vi "Staging1Wire.vi"() -> ()   [LabVIEW 2013]
uses:
  Device Driver/1WireSystem/subVis/position_TypDef.ctl
  shared programs/GUI_Template/GUI_master/tcp new data cluster.ctl
panel:
  in  "Position.Channel 8::1":T1(ring) caption="Position.Channel 7::1"
  in  "Filpper.Channel 8.Name::1":string caption="Filpper.Channel 7.Name::1"
  in  "Position.Channel 1::1":T2
  in  "all out":bool
  in  "Beam1":bool
  in  "Beam2":bool
  in  "Filpper.Channel 7.Name::1":string
  in  "Position.Channel 7::1":T1(ring)
  in  "Position.Channel 6::1":T1(ring)
  in  "Filpper.Channel 6.Name::1":string
  in  "Position.Channel 5::1":T1(ring)
  in  "Filpper.Channel 5.Name::1":string="Beam2 Near"
  in  "Position.Channel 4::1":T1(ring)
  in  "Filpper.Channel 4.Name::1":string="Beam1 Far"
  in  "Filpper.Channel 3.Name::1":string="Beam1 Near"
  in  "Filpper.Channel 2.Name::1":string="Beam2 Far"
  in  "Position.Channel 3::1":T1(ring)
  in  "Filpper.Channel 1.Name::1":string="XH1"
  in  "Position.Channel 2::1":T1(ring)
  out "device status::1":string="Initialized"
  in  "stop":bool
  in  "GUIdevice 1":string="Staging1Wire"
  out "UDP error message":string
  in  "insert tag":bool=TRUE
  # "Staging 1Wire"
  # "Far"
  # "Near"
  # "Far"
  # "Near"
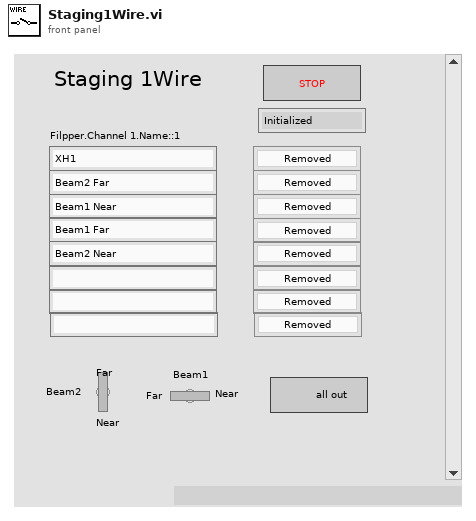
[diagram p1: front panel]
types:
  T1 = enum16{"Removed", "Inserted", "Unknown", "Moving"}
  T2 = typedef "position_TypDef.ctl" = enum16{"Removed", "Inserted", "Unknown", "Moving"}
  T3 = typedef "tcp new data cluster.ctl" = cluster{"EventEnum":enum16{"new data", "connection status update"}, "Device name":string}
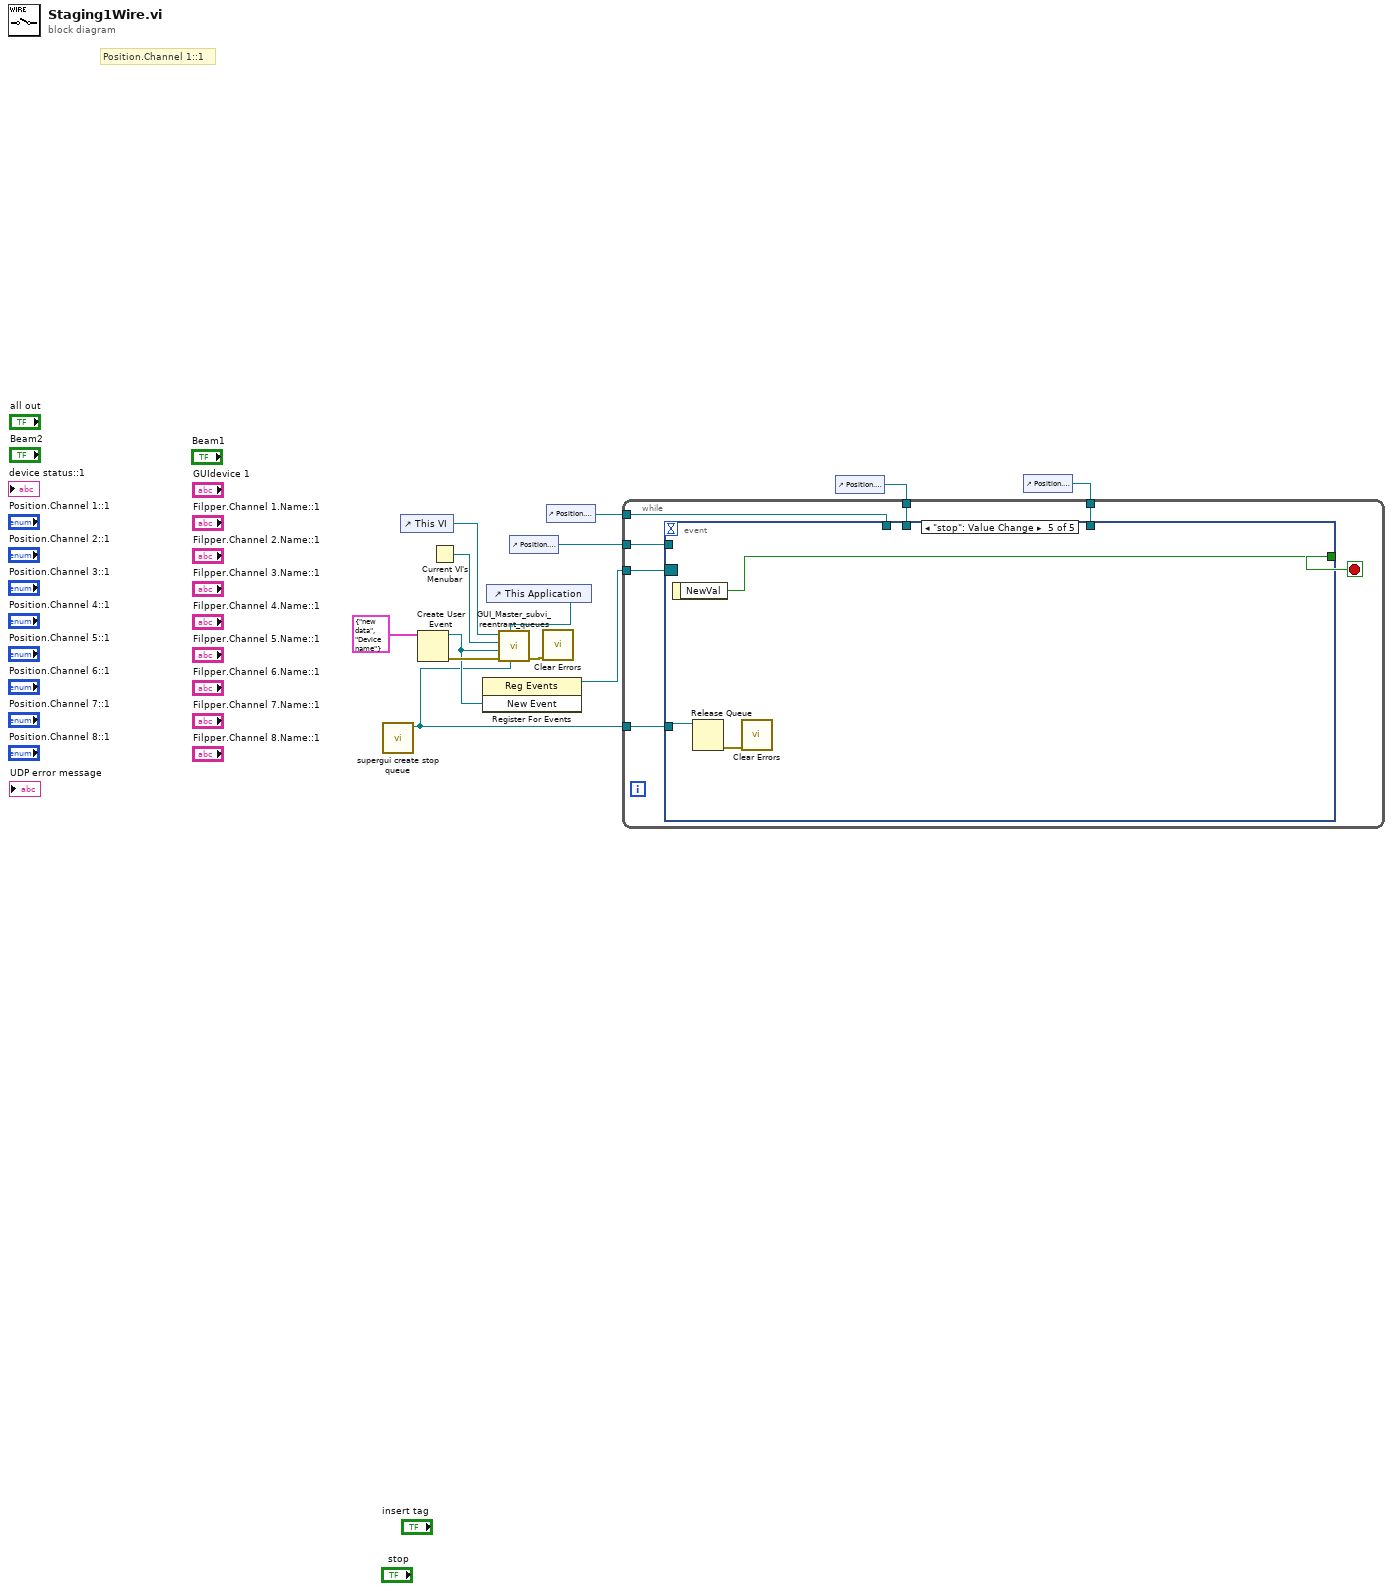
[diagram p0: block diagram]
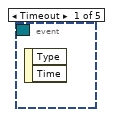
[diagram p2: hidden frame]
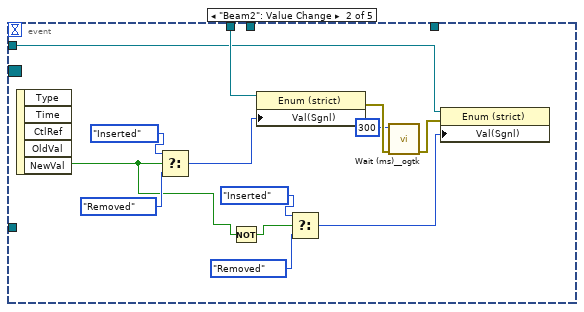
[diagram p3: hidden frame]
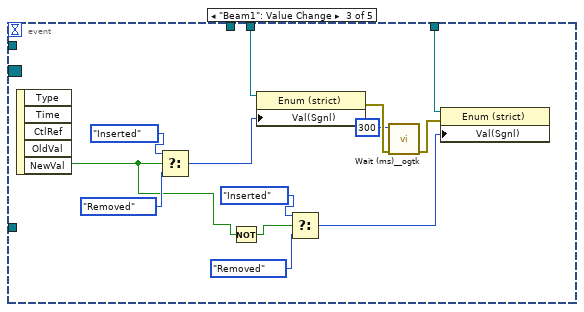
[diagram p4: hidden frame]
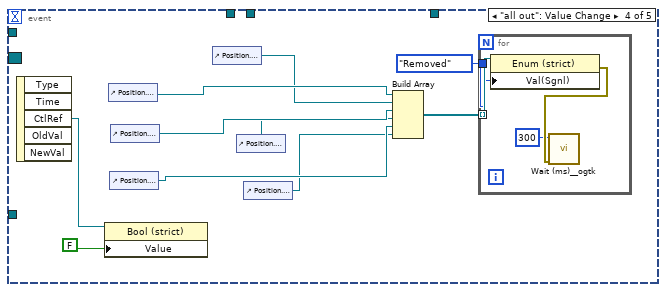
[diagram p5: hidden frame]
diagram:
  # "Position.Channel 1::1"
  n1 = call "supergui create stop queue.vi"() -> ("STOP Queue out"=w1:refnum<queue>)  [unwired: 11 in]
  n2 = control-ref of="This VI"() -> (w13:refnum<vi>)
  n3 = Create User Event(user event datatype=T3 {"EventEnum"=enum."new data", "Device name"="Device name"} ("New Event")) -> (user event=w8:refnum<user-event>, error out=w10:errorcluster)  [unwired: 1 in]
  n4 = Current VI's Menubar() -> (w12:refnum<k9>)
  n5 = register-events(w8) -> (reference out=w7:refnum<event-registration>)  [unwired: 2 in, 1 out]
  n6 = control-ref of="This Application"() -> (w2:refnum<vi>)
  n7 = call "GUI_Master_subvi_reentrant_queues.vi"("STOP Queue in"=w1, "This Application"=w2, "error in (no error)"=w10, "tcp data event"=w8, "Caller menu reference"=w12, "Caller VI ref"=w13) -> ("error out"=w9:errorcluster)  [unwired: 5 in]
  n8 = control-ref of="Position.Channel 5::1"() -> (w5:refnum<vi>)
  n9 = call <vilib>:"Clear Errors.vi"("error in (no error)"=w9) -> ()  [unwired: 6 in, 1 out]
  n10 = control-ref of="Position.Channel 2::1"() -> (w6:refnum<vi>)
  n11 = control-ref of="Position.Channel 3::1"() -> (w4:refnum<vi>)
  n12 = control-ref of="Position.Channel 4::1"() -> (w3:refnum<vi>)
  n13 = while {
    tunnel: w7 -> [w20]
    tunnel: w6 -> [w18]
    tunnel: w5 -> [w17]
    tunnel: w4 -> [w16]
    tunnel: w3 -> [w15]
    tunnel: w1 -> [w14]
    stop <- w19 stop-if-true
    n14 = event shown="[4] \"stop\": Value Change" {
      selector: w20 -> [_ _ _ _ _]
      dyn-events: _ -> [_ _ _ _ _]
      timeout: _ -> [_ _ _ _ _]
      tunnel: [_ _ _ _ w63] -> w19
      tunnel: w18 -> [_ w33 _ _ _]
      tunnel: w17 -> [_ w26 _ _ _]
      tunnel: w16 -> [_ _ w35 _ _]
      tunnel: w15 -> [_ _ w34 _ _]
      tunnel: w14 -> [_ _ _ _ w62]
      event Timeout {
        n15 = event-data() -> ()  [unwired: 1 in, 2 out]
      }
      event "Beam2": Value Change {
        n16 = event-data() -> ("NewVal"=w28:bool)  [unwired: 1 in, 4 out]
        n17 = Select(t=T1."Inserted" ("Value"), s=w28, f=T1."Removed" ("Value")) -> (s? t:f=w24:T1)
        n18 = Not(x=w28) -> (.not. x?=w27:bool)
        n19 = property class="Enum (strict)"(reference=w33, "Val(Sgnl)"=w24) -> (error out=w23:errorcluster)  [unwired: 1 in, 1 out]
        n20 = Select(t=T1."Inserted" ("Value"), s=w27, f=T1."Removed" ("Value")) -> (s? t:f=w25:T1)
        n21 = call <userlib>:"Wait (ms)__ogtk.vi"("error in (no error)"=w23, "milliseconds to wait"=u32 300) -> ("error out"=w22:errorcluster)  [unwired: 8 in, 1 out]
        n22 = property class="Enum (strict)"(reference=w26, error in=w22, "Val(Sgnl)"=w25) -> ()  [unwired: 2 out]
      }
      event "Beam1": Value Change {
        n23 = event-data() -> ("NewVal"=w42:bool)  [unwired: 1 in, 4 out]
        n24 = Select(t=T1."Inserted" ("Value"), s=w42, f=T1."Removed" ("Value")) -> (s? t:f=w39:T1)
        n25 = Not(x=w42) -> (.not. x?=w41:bool)
        n26 = property class="Enum (strict)"(reference=w35, "Val(Sgnl)"=w39) -> (error out=w38:errorcluster)  [unwired: 1 in, 1 out]
        n27 = Select(t=T1."Inserted" ("Value"), s=w41, f=T1."Removed" ("Value")) -> (s? t:f=w40:T1)
        n28 = call <userlib>:"Wait (ms)__ogtk.vi"("error in (no error)"=w38, "milliseconds to wait"=u32 300) -> ("error out"=w37:errorcluster)  [unwired: 8 in, 1 out]
        n29 = property class="Enum (strict)"(reference=w34, error in=w37, "Val(Sgnl)"=w40) -> ()  [unwired: 2 out]
      }
      event "all out": Value Change {
        n30 = event-data() -> ("CtlRef"=w49:refnum<vi>)  [unwired: 1 in, 4 out]
        n31 = property class="Bool (strict)"(reference=w49, "Value"=FALSE) -> ()  [unwired: 1 in, 2 out]
        n32 = control-ref of="Position.Channel 5::1"() -> (w56:refnum<vi>)
        n33 = control-ref of="Position.Channel 7::1"() -> (w53:refnum<vi>)
        n34 = control-ref of="Position.Channel 6::1"() -> (w55:refnum<vi>)
        n35 = control-ref of="Position.Channel 1::1"() -> (w47:refnum<vi>)
        n36 = control-ref of="Position.Channel 2::1"() -> (w54:refnum<vi>)
        n37 = control-ref of="Position.Channel 3::1"() -> (w52:refnum<vi>)
        n38 = Build Array(w56, w47, w55, w54, w53, w52) -> (w51:refnum<vi>[])
        n39 = for {
          tunnel: w51 -> [w60] mode=indexing
          tunnel: T1."Removed" ("Value") -> [w59]
          n40 = property class="Enum (strict)"(reference=w60, "Val(Sgnl)"=w59) -> (error out=w58:errorcluster)  [unwired: 1 in, 1 out]
          n41 = call <userlib>:"Wait (ms)__ogtk.vi"("error in (no error)"=w58, "milliseconds to wait"=u32 300) -> ()  [unwired: 8 in, 2 out]
        }
      }
      event "stop": Value Change {
        n42 = event-data() -> ("NewVal"=w63:bool)  [unwired: 1 in]
        n43 = Release Queue(queue=w62) -> (error out=w61:errorcluster)  [unwired: 2 in, 2 out]
        n44 = call <vilib>:"Clear Errors.vi"("error in (no error)"=w61) -> ()  [unwired: 6 in, 1 out]
      }
    }
  }
